vi "Start.vi"(8 "error in (no error)":errorcluster, 11 "Module Config Selector":i16) -> (0 "error out":errorcluster)   [LabVIEW 2017, in "BOP_VibAPI_6.lvlib"]
uses:
  <vilib>/addons/InsightCM/Devices/Shared/Cms/Fpga/Acquisition/source/subVIs/VibAPI/BOP_VibAPI_6.lvlib
  <vilib>/rvi/eio/common/nirviEmuTemplateMethod_errors.vi
  <vilib>/eio/EIONode/EIONode.xnode
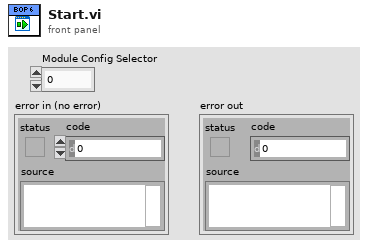
[diagram p1: front panel]
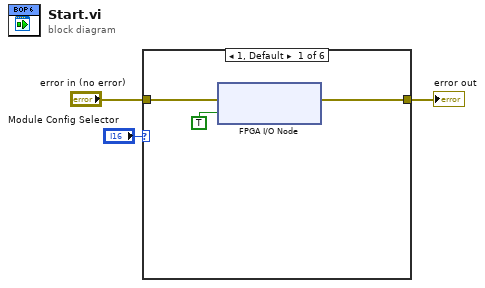
[diagram p0: block diagram]
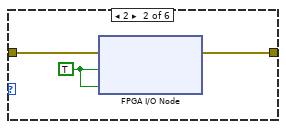
[diagram p2: hidden frame]
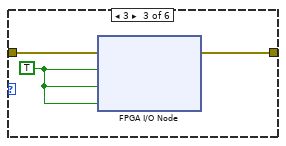
[diagram p3: hidden frame]
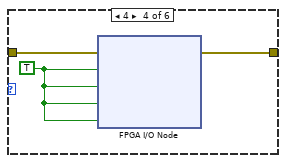
[diagram p4: hidden frame]
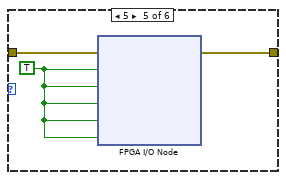
[diagram p5: hidden frame]
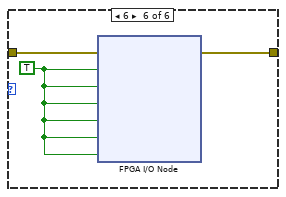
[diagram p6: hidden frame]
diagram:
  n1 = case shown="1, Default" "Module Config Selector" {
    tunnel: "error in (no error)" -> [w5 w8 w12 w15 w18 w21]
    tunnel: [w6 w9 w10 w14 w17 w20] -> w2
    frame 1, Default {
      n2 = xnode "FPGA I/O Node"("error in"=w5, "Mod1/Start"=TRUE) -> ("error out"=w6:errorcluster)  [unwired: 1 in, 1 out]
    }
    frame 2 {
      w7 = TRUE
      n3 = xnode "FPGA I/O Node"("error in"=w8, "Mod1/Start"=w7, "Mod2/Start"=w7) -> ("error out"=w9:errorcluster)  [unwired: 2 in, 2 out]
    }
    frame 3 {
      w11 = TRUE ("Mod1/Start")
      n4 = xnode "FPGA I/O Node"("error in"=w12, "Mod1/Start"=w11, "Mod2/Start"=w11, "Mod3/Start"=w11) -> ("error out"=w10:errorcluster)  [unwired: 3 in, 3 out]
    }
    frame 4 {
      w13 = TRUE ("Mod1/Start")
      n5 = xnode "FPGA I/O Node"("error in"=w15, "Mod1/Start"=w13, "Mod2/Start"=w13, "Mod3/Start"=w13, "Mod4/Start"=w13) -> ("error out"=w14:errorcluster)  [unwired: 4 in, 4 out]
    }
    frame 5 {
      w16 = TRUE ("Mod1/Start")
      n6 = xnode "FPGA I/O Node"("error in"=w18, "Mod1/Start"=w16, "Mod2/Start"=w16, "Mod3/Start"=w16, "Mod4/Start"=w16, "Mod5/Start"=w16) -> ("error out"=w17:errorcluster)  [unwired: 5 in, 5 out]
    }
    frame 6 {
      w19 = TRUE ("Mod1/Start")
      n7 = xnode "FPGA I/O Node"("error in"=w21, "Mod1/Start"=w19, "Mod2/Start"=w19, "Mod3/Start"=w19, "Mod4/Start"=w19, "Mod5/Start"=w19, "Mod6/Start"=w19) -> ("error out"=w20:errorcluster)  [unwired: 6 in, 6 out]
    }
  }
  "error out" <- w2
